vi "FVIR_LDO_Agilent_34972A-Convert Resistance.vi"(8 "error in (no error)":errorcluster, 10 "Output Array":dbl[](array[numeric])) -> (0 "error out":errorcluster, 1 "Agilent Data":T1)   [LabVIEW 2023]
uses:
  Agilent Data.ctl
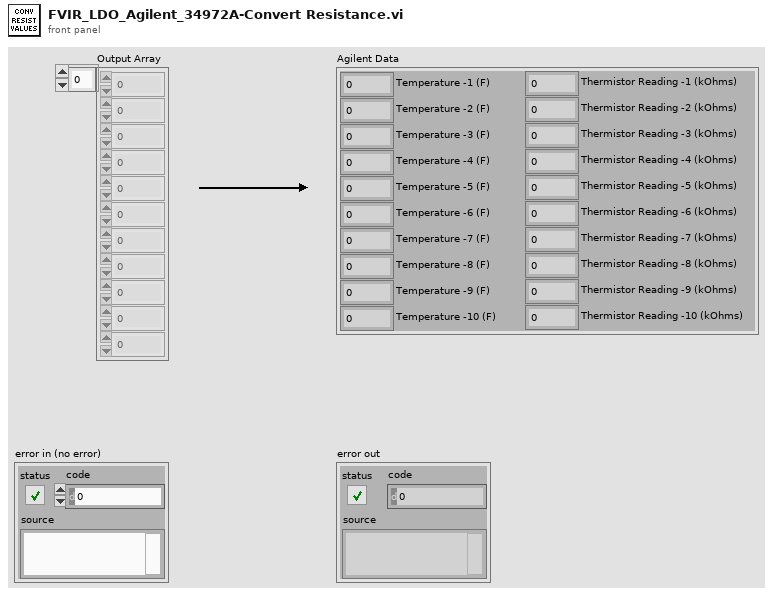
[diagram p1: front panel]
types:
  T1 = typedef "Agilent Data.ctl" = cluster{"Temperature -1 (F)":dbl, "Thermistor Reading -1 (kOhms)":dbl, "Thermistor Reading -2 (kOhms)":dbl, "Temperature -2 (F)":dbl, "Thermistor Reading -3 (kOhms)":dbl, "Temperature -3 (F)":dbl, "Thermistor Reading -4 (kOhms)":dbl, "Temperature -4 (F)":dbl, "Thermistor Reading -5 (kOhms)":dbl, "Temperature -5 (F)":dbl, "Thermistor Reading -6 (kOhms)":dbl, "Temperature -6 (F)":dbl, "Thermistor Reading -7 (kOhms)":dbl, "Temperature -7 (F)":dbl, "Thermistor Reading -8 (kOhms)":dbl, "Temperature -8 (F)":dbl, "Thermistor Reading -9 (kOhms)":dbl, "Temperature -9 (F)":dbl, "Thermistor Reading -10 (kOhms)":dbl, "Temperature -10 (F)":dbl}
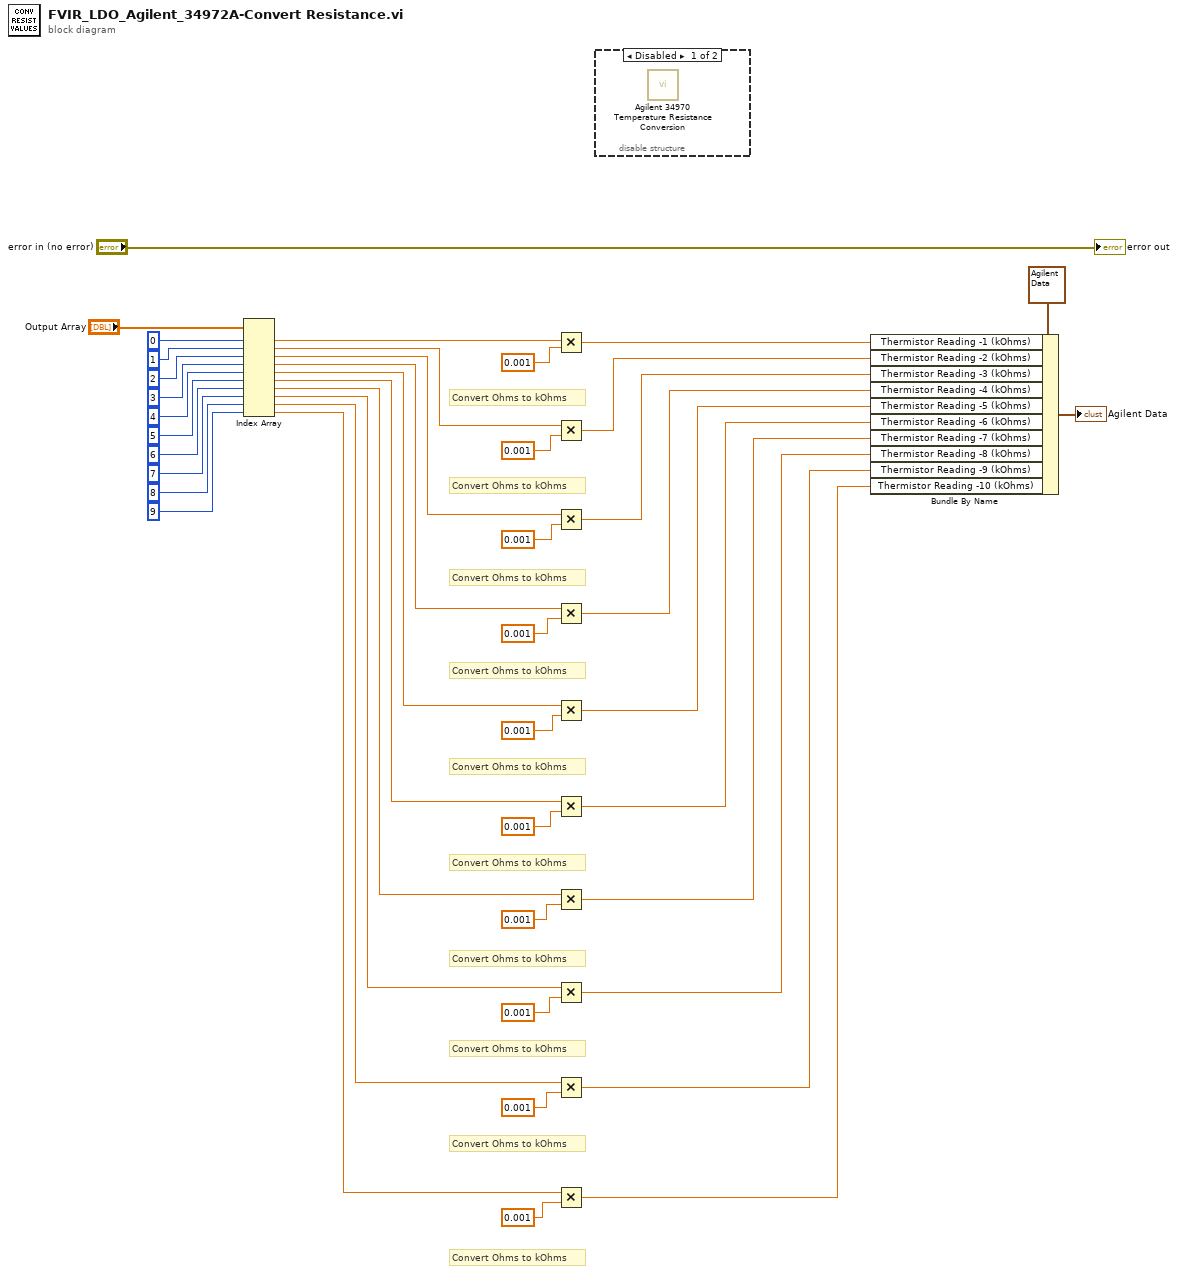
[diagram p0: block diagram]
diagram:
  # "Convert Ohms to kOhms"
  # "Convert Ohms to kOhms"
  # "Convert Ohms to kOhms"
  # "Convert Ohms to kOhms"
  # "Convert Ohms to kOhms"
  # "Convert Ohms to kOhms"
  # "Convert Ohms to kOhms"
  # "Convert Ohms to kOhms"
  # "Convert Ohms to kOhms"
  # "Convert Ohms to kOhms"
  n1 = Index Array(array="Output Array", index #1=0 ("index"), index #2=1 ("index"), index #3=2 ("index"), index #4=3 ("index"), index #5=4 ("index"), index #6=5 ("index"), index #7=6 ("index"), index #8=7 ("index"), index #9=8 ("index"), index #10=9 ("index")) -> (element #1=w39:dbl, element #2=w19:dbl, element #3=w18:dbl, element #4=w17:dbl, element #5=w16:dbl, element #6=w15:dbl, element #7=w14:dbl, element #8=w13:dbl, element #9=w12:dbl, element #10=w11:dbl)
  n2 = Multiply(x=w39, y=0.001) -> (x*y=w43:dbl)
  n3 = Multiply(x=w19, y=0.001) -> (x*y=w10:dbl)
  n4 = Multiply(x=w18, y=0.001) -> (x*y=w9:dbl)
  n5 = Multiply(x=w17, y=0.001) -> (x*y=w8:dbl)
  n6 = Multiply(x=w16, y=0.001) -> (x*y=w7:dbl)
  n7 = Multiply(x=w15, y=0.001) -> (x*y=w6:dbl)
  n8 = Multiply(x=w14, y=0.001) -> (x*y=w5:dbl)
  n9 = Multiply(x=w13, y=0.001) -> (x*y=w4:dbl)
  n10 = Multiply(x=w12, y=0.001) -> (x*y=w3:dbl)
  n11 = Multiply(x=w11, y=0.001) -> (x*y=w2:dbl)
  n12 = disable-structure shown="Disabled" {
    frame Disabled {
      n13 = call "Agilent 34970 Temperature Resistance Conversion.vi"() -> ()  [unwired: 10 in, 2 out]
    }
    frame Enabled {
    }
  }
  n14 = Bundle By Name(cluster=T1 {"Temperature -1 (F)"=0.0, "Thermistor Reading -1 (kOhms)"=0.0, "Thermistor Reading -2 (kOhms)"=0.0, "Temperature -2 (F)"=0.0, "Thermistor Reading -3 (kOhms)"=0.0, "Temperature -3 (F)"=0.0, "Thermistor Reading -4 (kOhms)"=0.0, "Temperature -4 (F)"=0.0, "Thermistor Reading -5 (kOhms)"=0.0, "Temperature -5 (F)"=0.0, "Thermistor Reading -6 (kOhms)"=0.0, "Temperature -6 (F)"=0.0, "Thermistor Reading -7 (kOhms)"=0.0, "Temperature -7 (F)"=0.0, "Thermistor Reading -8 (kOhms)"=0.0, "Temperature -8 (F)"=0.0, "Thermistor Reading -9 (kOhms)"=0.0, "Temperature -9 (F)"=0.0, "Thermistor Reading -10 (kOhms)"=0.0, "Temperature -10 (F)"=0.0}, "Thermistor Reading -1 (kOhms)"=w43, "Thermistor Reading -2 (kOhms)"=w10, "Thermistor Reading -3 (kOhms)"=w9, "Thermistor Reading -4 (kOhms)"=w8, "Thermistor Reading -5 (kOhms)"=w7, "Thermistor Reading -6 (kOhms)"=w6, "Thermistor Reading -7 (kOhms)"=w5, "Thermistor Reading -8 (kOhms)"=w4, "Thermistor Reading -9 (kOhms)"=w3, "Thermistor Reading -10 (kOhms)"=w2) -> (→"Agilent Data":T1)
  "error out" <- "error in (no error)"
